vi "Set Static (Func Global).vi"(8 "error in (no error)":errorcluster, 10 "Int":i32, 11 "Numeric in":refnum<class "Numeric Test Object.lvclass">) -> (0 "error out":errorcluster, 3 "Numeric out":refnum<class "Numeric Test Object.lvclass">)   [LabVIEW 2009, in "Numeric Test Object.lvclass"]
doc: "Sets the data held by the functional global vi."
uses:
  Numeric Test Object.lvclass
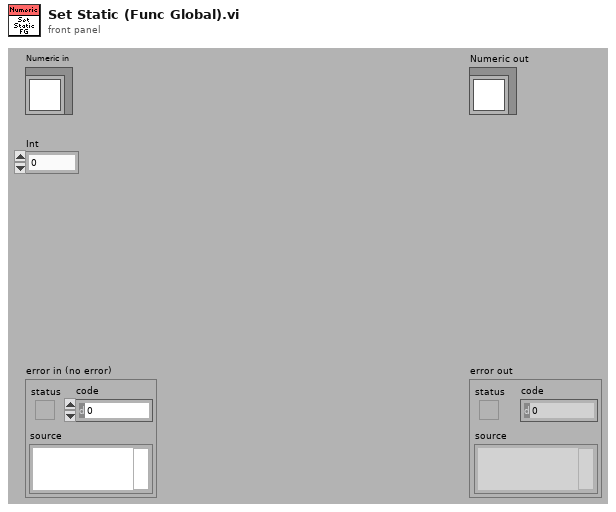
[diagram p1: front panel]
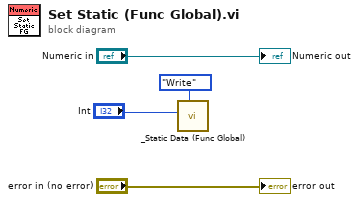
[diagram p0: block diagram]
diagram:
  n1 = call "_Static Data (Func Global).vi"("Function (Read)"=enum16{"Read", "Write"}."Write", "Numeric (0)"="Int") -> ()  [unwired: 7 in, 3 out]
  "error out" <- "error in (no error)"
  "Numeric out" <- "Numeric in"
